vi "VI Is Running.vi"(8 "error in (no error)":errorcluster, 11 "VI in":refnum<vi>) -> (0 "error out":errorcluster, 2 "Running?":bool, 3 "VI out":refnum<vi>)   [LabVIEW 2014, in "UI_ProgressDlg.lvlib" / "UI_ProgressDlg.lvclass"]
uses:
  UI_ProgressDlg.lvclass
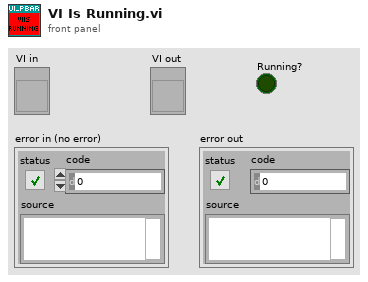
[diagram p1: front panel]
types:
  T1 = enum32{"Bad", "Idle", "Run top level", "Running"}
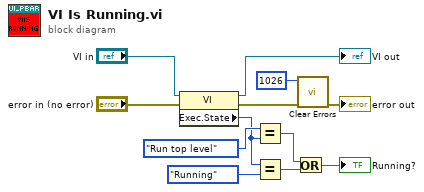
[diagram p0: block diagram]
diagram:
  n1 = property on="Property Node" class="VI"(reference="VI in", error in="error in (no error)") -> (reference out=→"VI out":refnum<vi>, error out=w3:errorcluster, "Exec.State"=w8:T1)
  n2 = Equal?(x=T1."Run top level" ("Execution:State"), y=w8) -> (x = y?=w6:bool)
  n3 = Equal?(x=w8, y=T1."Running" ("Execution:State")) -> (x = y?=w5:bool)
  n4 = Or(x=w6, y=w5) -> (x .or. y?=→"Running?":bool)
  n5 = call <vilib>:"Clear Errors.vi"("error in (no error)"=w3, "specific error code to clear (0: all)"=1026) -> ("error out"=→"error out":errorcluster)  [unwired: 4 in, 1 out]
